vi "Type Def.vi"(8 "error in (no error)":errorcluster, 10 "vi name":string, 11 "application reference":refnum<vi>) -> (0 "error out":errorcluster)   [LabVIEW 2020, in "Lazyboots Menu Tool Launch.lvlib"]
doc: "This is a type defined VI for dynamical call in menu VIs."
uses:
  _Library/Lazyboots Menu Tool Launch.lvlib
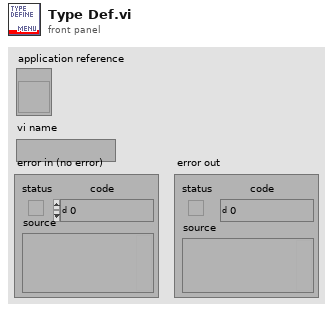
[diagram p1: front panel]
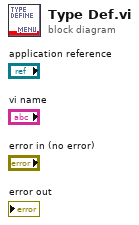
[diagram p0: block diagram]
diagram:
